vi "Scaled Time Domain Window (DBL).vi"(9 "window parameter":dbl=nan, 10 "window":T1 items=["Rectangle"=0, "Hanning"=1, "Hamming"=2, "Blackman-Harris"=3, "Exact Blackman"=4, "Blackman"=5, "Flat Top"=6, "4 Term B-Harris "=7, "7 Term B-Harris"=8, "Low Sidelobe"=9, "Blackman Nuttall"=11, "Triangle"=30, "Bartlett-Hanning"=31, "Bohman"=32, "Parzen"=33, "Welch"=34, "Kaiser"=60, "Dolph-Chebyshev"=61, "Gaussian"=62], 11 "X":dbl[](array[numeric])) -> (0 "error":i32, 2 "window properties":cluster{"eq noise BW":dbl, "coherent gain":dbl} {"coherent gain" format="%0.2f"; "eq noise BW" format="%0.2f"}, 3 "Windowed X":dbl[](array[numeric]))   [LabVIEW 2020, in "NI_AALPro.lvlib"]
doc: "Applies a scaled window to the input sequence <B>X</B>. Wire data to the <B>X</B> input to determine the polymorphic instance to use or manually select the instance."
uses:
  NI_AALPro.lvlib
  windowTd.ctl
  <resource>/lvanlys.dll
panel:
  # "Scaled Time Domain Window"
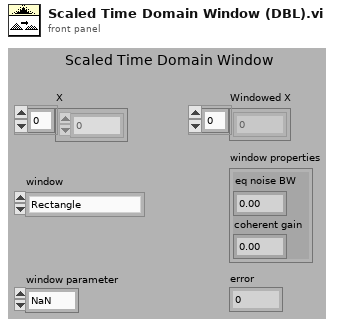
[diagram p1: front panel]
types:
  T1 = typedef "NI_AALPro.lvlib/windowTd.ctl" = u32
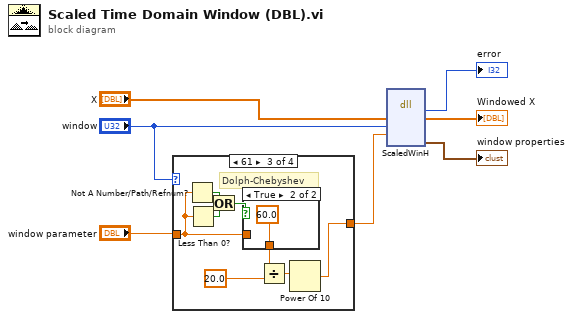
[diagram p0: block diagram]
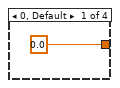
[diagram p2: hidden frame]
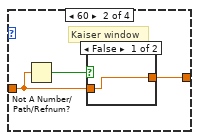
[diagram p3: hidden frame]
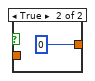
[diagram p4: hidden frame]
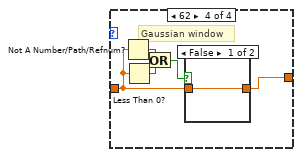
[diagram p6: hidden frame]
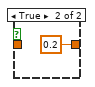
[diagram p7: hidden frame]
diagram:
  n1 = case shown="61" "window" {
    tunnel: [0.0 ("s(db)") w11 w19 w28] -> w1
    tunnel: "window parameter" -> [_ w10 w17 w26]
    frame 0, Default {
    }
    frame 60 {
      # "Kaiser window"
      n2 = Not A Number/Path/Refnum?(number/path/refnum=w10) -> (NaN/Path/Refnum?=w9:bool)
      n3 = case shown="False" w9 {
        tunnel: [w12 0] -> w11
        tunnel: w10 -> [w12 _]
        frame False {
        }
        frame True {
        }
      }
    }
    frame 61 {
      # "Dolph-Chebyshev"
      n4 = Not A Number/Path/Refnum?(number/path/refnum=w17) -> (NaN/Path/Refnum?=w16:bool)
      n5 = Less Than 0?(x=w17) -> (x < 0?=w15:bool)
      n6 = Or(x=w16, y=w15) -> (x .or. y?=w14:bool)
      n7 = case shown="True" w14 {
        tunnel: [w22 60.0 ("y")] -> w18
        tunnel: w17 -> [w22 _]
        frame False {
        }
        frame True {
        }
      }
      n8 = Divide(x=w18, y=20.0) -> (x/y=w20:dbl)
      n9 = Power Of 10(x=w20) -> (10^x=w19:dbl)
    }
    frame 62 {
      # "Gaussian window"
      n10 = Not A Number/Path/Refnum?(number/path/refnum=w26) -> (NaN/Path/Refnum?=w27:bool)
      n11 = Less Than 0?(x=w26) -> (x < 0?=w25:bool)
      n12 = Or(x=w27, y=w25) -> (x .or. y?=w24:bool)
      n13 = case shown="False" w24 {
        tunnel: w26 -> [w29 _]
        tunnel: [w29 0.2 ("para")] -> w28
        frame False {
        }
        frame True {
        }
      }
    }
  }
  n14 = dll-call lib="C:/Program Files (x86)/National Instruments/LabVIEW 2020/resource/lvanlys.*" fn="ScaledWinH"("xH"="X", "winType"="window", "para"=w1) -> ("return type"=→"error":i32, "xH"=→"Windowed X":dbl[], "window properties"=→"window properties":cluster{"eq noise BW":dbl, "coherent gain":dbl})  [unwired: 6 in, 2 out]
